vi "Subscribe.vi"(8 "error in (no error)":errorcluster, 10 "Subscription Request":refnum<class "SubscriptionRequest.lvclass">, 11 "Mediator In":refnum<class "IMediator.lvclass">) -> (0 "error out":errorcluster, 3 "Mediator Out":refnum<class "IMediator.lvclass">)   [LabVIEW 2015, in "IMediator.lvlib" / "IMediator.lvclass"]
doc: "<License>\nCopyright © 2017 Composed Systems, LLC | All rights reserved\nwww.composed.io\n\nAuthor: Ethan Stern <ethan.stern@composed.io>\n\nThis software is provided \"AS IS\" WITHOUT WARRANTIES, either express or implied, AND IS FOR EDUCATIONAL PURPOSES ONLY.\n</License>"
uses:
  IMediator.lvclass
  SubscriptionRequest/SubscriptionRequest.lvclass
panel:
  # "Who wants it?\nWhat do they want?\nWhat type are they expecting?\nHow do they want it sent?"
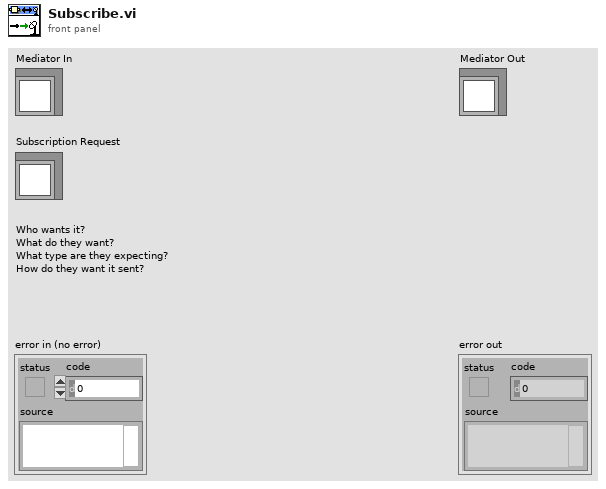
[diagram p1: front panel]
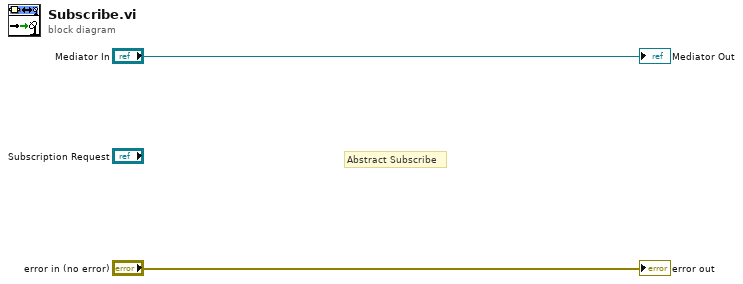
[diagram p0: block diagram]
diagram:
  # "Abstract Subscribe"
  "error out" <- "error in (no error)"
  "Mediator Out" <- "Mediator In"
